vi "commandSet (SubVI).vi"() -> (2 "CommandSet":string[](array[string]))   [LabVIEW 2019]
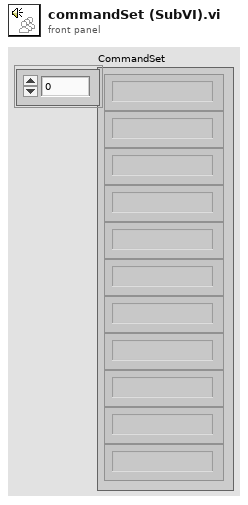
[diagram p1: front panel]
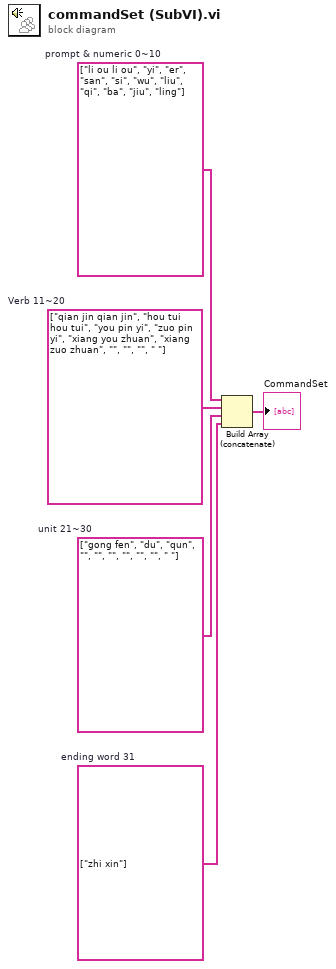
[diagram p0: block diagram]
diagram:
  w5 = string[] ["zhi xin"]  # ending word 31
  w4 = string[] ["gong fen", "du", "qun", "", "", "", "", "", "", " "]  # unit 21~30
  w3 = string[] ["qian jin qian jin", "hou tui hou tui", "you pin yi", "zuo pin yi", "xiang you zhuan", "xiang zuo zhuan", "", "", "", " "]  # Verb 11~20
  w1 = string[] ["li ou li ou", "yi", "er", "san", "si", "wu", "liu", "qi", "ba", "jiu", "ling"]  # prompt & numeric 0~10
  n1 = Build Array (concatenate)(w1, w3, w4, w5) -> (→"CommandSet":string[])
